vi "Fdx Create Monitor Queue.vi"(6 "RecordingFileName":path, 8 "error in (no error)":errorcluster, 9 "MaxFileSize MB (1)":u32=1, 11 "InstrumentHandle_port in":u32) -> (0 "error out":errorcluster, 1 "GlobMonSize":u32, 2 "QueueIdOut":u32, 3 "InstrumentHandle_port out":u32)   [LabVIEW 2020, in "AIM664LV.lvlib"]
uses:
  AIM664LV.lvlib
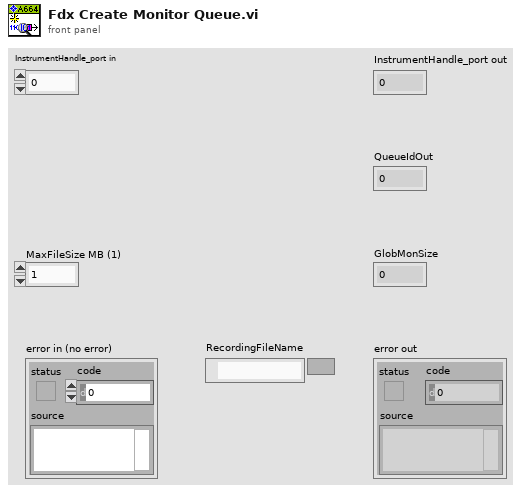
[diagram p1: front panel]
types:
  T1 = cluster{"QueueCtrl":u32, "QueueId":u32, "RecordingFileName":string, "MaxFileSize":u32}
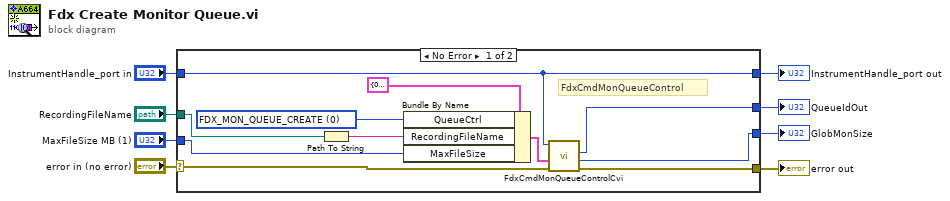
[diagram p0: block diagram]
diagram:
  n1 = case shown="No Error" "error in (no error)" {
    selector: "error in (no error)" -> [w19 w20]
    tunnel: "InstrumentHandle_port in" -> [w11 w21]
    tunnel: [w18 w20] -> w6
    tunnel: [w11 w21] -> w5
    tunnel: "MaxFileSize MB (1)" -> [w14 _]
    tunnel: "RecordingFileName" -> [w13 _]
    tunnel: [w10 _] -> w2
    tunnel: [w9 _] -> w1
    frame No Error {
      w15 = u32 0 items=["FDX_MON_QUEUE_CREATE", "FDX_MON_QUEUE_DELETE"] ("QueueCtrl")
      # "FdxCmdMonQueueControl"
      n2 = Path To String(path=w13) -> (string=w12:string)
      n3 = Bundle By Name(cluster=T1 {"QueueCtrl"=0, "QueueId"=0, "RecordingFileName"="", "MaxFileSize"=0} ("Q Ctrl In"), "QueueCtrl"=w15, "RecordingFileName"=w12, "MaxFileSize"=w14) -> (w16:T1)
      n4 = call "FdxCmdMonQueueControlCvi.vi"("error in"=w19, "Q Ctrl In"=w16, "InstrumentHandle_port"=w11) -> ("error out"=w18:errorcluster, "GlobMonSize"=w9:u32, "QueueIdOut"=w10:u32)  [unwired: 5 in, 1 out]
    }
    frame Error {
    }
  }
  "error out" <- w6
  "InstrumentHandle_port out" <- w5
  "GlobMonSize" <- w1
  "QueueIdOut" <- w2
